vi "Do.vi"(8 "error in (no error)":errorcluster, 10 "Actor in":refnum<class "Actor.lvclass">, 11 "Configure AC Bandwidth [AC] Msg":refnum<class "Configure AC Bandwidth [AC] Msg.lvclass">) -> (0 "error out":errorcluster, 2 "Actor out":refnum<class "Actor.lvclass">)   [LabVIEW 2015, in "CS++DMM.lvlib" / "Configure AC Bandwidth [AC] Msg.lvclass"]
doc: "This VI delivers the message to the actor by calling the appropriate method(s) on the actor."
uses:
  Configure AC Bandwidth [AC] Msg.lvclass
  <vilib>/ActorFramework/Actor/Actor.lvclass
  CS++DMM/CS++DMM.lvclass
  Configure AC Bandwidth [AC] Msg.lvclass/Configure AC Bandwidth [AC] Msg.ctl
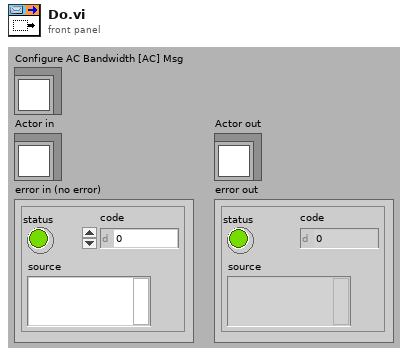
[diagram p1: front panel]
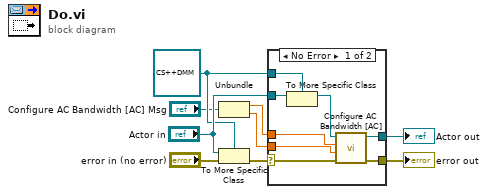
[diagram p0: block diagram]
diagram:
  w4 = refnum<class "CS++DMM.lvclass"> refnum ("Actor in")
  n1 = Unbundle ("Main-Unbundle")("Configure AC Bandwidth [AC] Msg") -> (w2:dbl, w1:dbl)
  n2 = To More Specific Class(target class=w4, reference="Actor in", error in="error in (no error)") -> (error out=w8:errorcluster)  [unwired: 1 out]
  n3 = case shown="No Error" w8 {
    selector: w8 -> [w15 w19]
    tunnel: [w17 w19] -> w7
    tunnel: [w16 w18] -> w6
    tunnel: "Actor in" -> [w14 w18]
    tunnel: w4 -> [w13 _]
    tunnel: w2 -> [w11 _]
    tunnel: w1 -> [w10 _]
    frame No Error {
      n4 = To More Specific Class(target class=w13, reference=w14) -> (specific class reference=w12:refnum<class "CS++DMM.lvclass">)  [unwired: 1 in, 1 out]
      n5 = call "Configure AC Bandwidth [AC].vi"("error in (no error)"=w15, "ac max frequency (300.0E+3 Hz)"=w10, "ac min frequency (20.0 Hz)"=w11, "CS++DMM in"=w12) -> ("error out"=w17:errorcluster, "CS++DMM out"=w16:refnum<class "CS++DMM.lvclass">)  [unwired: 6 in]
    }
    frame Error {
    }
  }
  "error out" <- w7
  "Actor out" <- w6
